vi "Untitled 1.vi"(8 "error in (no error)":errorcluster, 11 "MARLIN in":refnum<class "MARLIN.lvclass">) -> (0 "error out":errorcluster, 3 "MARLIN out":refnum<class "MARLIN.lvclass">)   [LabVIEW 2017, in "MARLIN.lvclass"]
uses:
  MARLIN.lvclass
  MARLIN.lvclass/MARLIN.ctl
panel:
  in  "Numeric":dbl
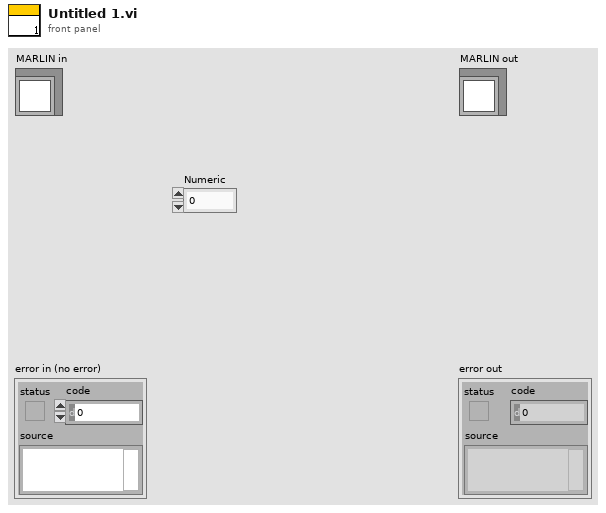
[diagram p1: front panel]
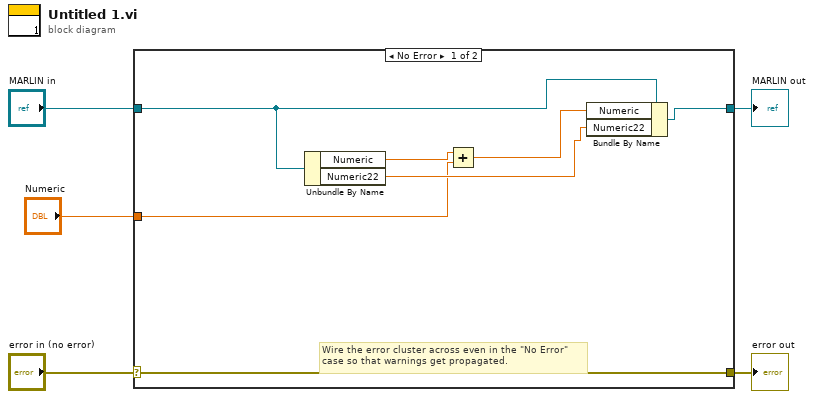
[diagram p0: block diagram]
diagram:
  n1 = case shown="No Error" "error in (no error)" {
    selector: "error in (no error)" -> [w12 w14]
    tunnel: [w12 w14] -> w4
    tunnel: [w7 w13] -> w2
    tunnel: "MARLIN in" -> [w10 w13]
    tunnel: "Numeric" -> [w6 _]
    frame No Error {
      # "Wire the error cluster across even in the \"No Error\"\ncase so that warnings get propagated."
      n2 = Unbundle By Name(w10) -> ("Numeric"=w11:dbl, "Numeric22"=w8:dbl)
      n3 = Add(x=w11, y=w6) -> (x+y=w9:dbl)
      n4 = Bundle By Name(cluster=w10, "Numeric"=w9, "Numeric22"=w8) -> (w7:refnum<class "MARLIN.lvclass">)
    }
    frame Error {
    }
  }
  "error out" <- w4
  "MARLIN out" <- w2
